vi "TR_Repair_TDMS_track.vi"(8 "error in (no error)":errorcluster, 10 "Parameters":T1, 11 "TDMS track":path) -> (0 "error out":errorcluster)   [LabVIEW 2018, in "Tracks Repair.lvlib"]
uses:
  Tracks Repair.lvlib
  SubVi's/Controls/CTL_Overlays_cluster.ctl
  SubVi's/Controls/CTL_Settings_cluster.ctl
  SubVi's/Controls/CTL_Histogram_parameters.ctl
  SubVi's/Controls/CTL_Filter_selector.ctl
  SubVi's/Controls/CTL_Acquisition_speed_selector.ctl
  SubVi's/Controls/CTL_Segmented_plot_parameters.ctl
  SubVi's/Controls/CTL_IO_params_cluster.ctl
  SubVi's/Controls/CTL_Conditions_Array.ctl
  SubVi's/Controls/CTL_Conditions_Cluster.ctl
  SubVi's/Controls/CTL_Condition_type.ctl
  SubVi's/Controls/CTL_Comparison_type.ctl
  SubVi's/Controls/CTL_Validity_check_criteria.ctl
  SubVi's/Controls/CTL_Response_info.ctl
  SubVi's/Controls/CTL_Condition_response_type.ctl
  SubVi's/Controls/CTL_Reponse_port_info.ctl
  SubVi's/Controls/CTL_Calibration_parameters.ctl
  SubVi's/Controls/CTL_Dispenser_calibration_info.ctl
  SubVi's/Controls/CTL_Post-processing_params.ctl
  SubVi's/Controls/CTL_Mouse_Draw_Params.ctl
  <vilib>/vision/Image Controls.llb/IMAQ Image.ctl
  SubVi's/Controls/CTL_Pixel_to_Zone_array.ctl
  SubVi's/Controls/CTL_Basic_cage_settings.ctl
  <userlib>/_OpenG.lib/md5/md5.llb/MD5 Message Digest (Hexadecimal String)__ogtk.vi
  <userlib>/_OpenG.lib/file/file.llb/Strip Path Extension - String__ogtk.vi
  Tracker.lvlib
panel:
  in  "Decimate?":bool
  out "Overlays cluster out":T2
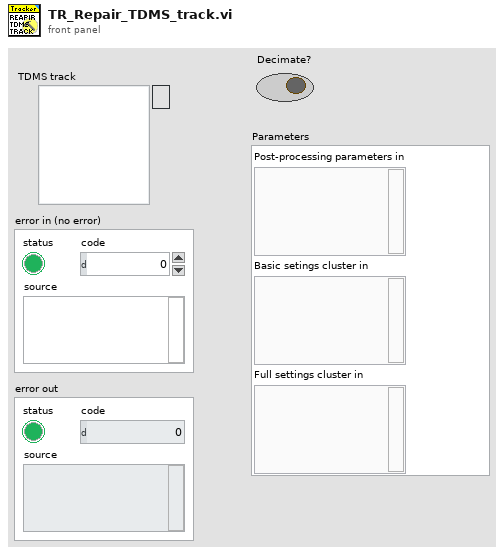
[diagram p1: front panel]
types:
  T1 = cluster{"Post-processing parameters in":variant, "Basic setings cluster in":variant, "Full settings cluster in":variant}
  T2 = typedef "Tracker.lvlib/CTL_Overlays_cluster.ctl" = cluster{"Time-coded track overlay (array)":u32[][], "Speed-coded track overlay (array)":u32[][], "Plain track overlay pixmap":u32[][], "Location density map image":u32[][], "Speed density map image":u32[][], "Location density map":dbl[][], "Speed density map":dbl[][]}
  T3 = enum16{"big-endian, network order", "native, host order", "little-endian"}
  T4 = enum16{"open", "open or create", "create or replace", "create", "open (read-only)"}
  T5 = typedef "Tracker.lvlib/CTL_Basic_cage_settings.ctl" = cluster{"Vert. offset":dbl, "Hor. offset":dbl, "Bridge swap":bool, "Twisted neck":bool, "Cage diam.":i32, "Magn.rot.":i32, "Acq. speed":dbl}
  T6 = typedef "Tracker.lvlib/CTL_Post-processing_params.ctl" = cluster{"Defragment TDMS? (F)":bool, "Start time (SW)":timestamp, "Start time (HW)":u32, "Data filtering":T7, "Mouse drawing parameters":T8, "Size of the image (480x480)":cluster{"X size":dbl, "Y size":dbl}, "Image ref. in":T9, "Calibration parameters":T10, "Pixel to zone":T12}
  T7 = typedef "Tracker.lvlib/CTL_Filter_selector.ctl" = cluster{"Filter type":enum16{"None", "Savitzky-Golay"}, "Length":i32, "Order":i32}
  T8 = typedef "Tracker.lvlib/CTL_Mouse_Draw_Params.ctl" = cluster{"Trace length, samples":u16, "Rainbow track":bool, "Rainbow track is speed":bool, "Bright mouse lineout":bool, "Colors array":u32[], "Pixels per mm":dbl}
  T9 = typedef "IMAQ Image.ctl" = refnum<image>
  T10 = typedef "Tracker.lvlib/CTL_Calibration_parameters.ctl" = cluster{"Timing calibration sw/hw":dbl, "True FPS":dbl, "True frame time, s":dbl, "Disp. calibration info":T11}
  T11 = typedef "Tracker.lvlib/CTL_Dispenser_calibration_info.ctl" = cluster{"Channel":u8, "Speed, µl per ms":dbl}[]
  T12 = typedef "Tracker.lvlib/CTL_Pixel_to_Zone_array.ctl" = i8[][]
  T13 = typedef "Tracker.lvlib/CTL_Settings_cluster.ctl" = cluster{"Defaults":cluster{"Default User":dbl, "VISA Resource Name ":string, "Histogram parameters":T14}, "Recording and saving":cluster{"Researcher name":string, "Name prefix":string, "Data post-processing":T7, "Stop at":dbl, "\"Stop at\" enabled":bool, "Default save folder path":path, "Acquisition FPS":T15}, "Geometry":T16, "IO parameters":T17, "Conditions presets array":T18, "Calibration parameters":T10, "Settings loaded OK":bool}
  T14 = typedef "Tracker.lvlib/CTL_Histogram_parameters.ctl" = cluster{"max":dbl, "min":dbl, "# bins":i32, "threshold":dbl, "thr. type":enum16{"higher accepted", "lower accepted"}}
  T15 = typedef "Tracker.lvlib/CTL_Acquisition_speed_selector.ctl" = enum16{"Max", "Optimal", "Eco"}
  T16 = typedef "Tracker.lvlib/CTL_Segmented_plot_parameters.ctl" = cluster{"Cage diameter, mm":u16, "Starting angle MIDFIELD":i16, "Starting angle BORDER":i16, "Radius, mm CENTER":u16, "Radius, mm MIDFIELD":u16, "N segments MIDFIELD":u8, "N segments BORDER":u8, "R-gap, mm":sgl, "Bridge swap":bool, "Bridge H. offset":sgl, "Bridge V. offset":sgl, "Twisted neck":bool, "Alt. magn. orientation":bool, "Sensor board size":enum16{"Small", "Large"}}
  T17 = typedef "Tracker.lvlib/CTL_IO_params_cluster.ctl" = cluster{"IO general config.":u16, "IO 1 configuration":u16, "IO 2 configuration":u16, "IO 3 configuration":u16, "IO 4 configuration":u16, "Activate ext. RS-232":u16, "IO inversion config.":u16, "Sync capability":u8}
  T18 = typedef "Tracker.lvlib/CTL_Conditions_Array.ctl" = T19[]
  T19 = typedef "Tracker.lvlib/CTL_Conditions_Cluster.ctl" = cluster{"Enabled":bool, "Name":string, "Specifier(s)":cluster{"Specifier enabled":bool, "Condition type":T20, "Comparison type":T21, "Value":dbl, "Validity criteria(s)":cluster{"V. check enabled":bool, "Criteria":T22, "Validity value":dbl}[]}[], "Response":T23, "Has been set":bool}
  T20 = typedef "Tracker.lvlib/CTL_Condition_type.ctl" = enum16{"Speed", "Zone", "Angle to wall"}
  T21 = typedef "Tracker.lvlib/CTL_Comparison_type.ctl" = enum16{"Less", "Less or Equal", "Equal", "Greater or Equal", "Greater", "Not Equal"}
  T22 = typedef "Tracker.lvlib/CTL_Validity_check_criteria.ctl" = enum16{"Running bout (seconds)", "Running bout (meters)"}
  T23 = typedef "Tracker.lvlib/CTL_Response_info.ctl" = cluster{"Response type":T24, "TTL port":T25, "TTL pulse length, ms":dbl}
  T24 = typedef "Tracker.lvlib/CTL_Condition_response_type.ctl" = enum16{"None", "Air puff", "Liquid reward"}
  T25 = typedef "Tracker.lvlib/CTL_Reponse_port_info.ctl" = enum16{"Port 1", "Port 2", "Port 3", "Port 4"}
  T26 = typedef "Tracker.lvlib/CTL_Cage_Coords_(arrays).ctl" = cluster{"R from center":dbl[], "sin(a)":dbl[], "Mouse Xc":dbl[], "Mouse Yc":dbl[], "X1-X2":dbl[], "Y1-Y2":dbl[], "Cage Xc":dbl[], "Cage Yc":dbl[], "Frame time, s":dbl}
  T27 = typedef "Tracker.lvlib/CTL_Animal_Coordinates_and_Speed_(arr).ctl" = cluster{"R from center":dbl[], "phi (mouse angular position in the cage)":dbl[], "alpha (mouse rot. angle)":dbl[], "X":dbl[], "Y":dbl[], "theta (from center towards mouse)":dbl[], "beta (cage rot. against mouse)":dbl[], "w (mouse angle to wall)":dbl[], "Speed (filtered)":dbl[], "Zone":i8[]}
  T28 = cluster{"Boolean Round":bool, "code":i32, "source":string}
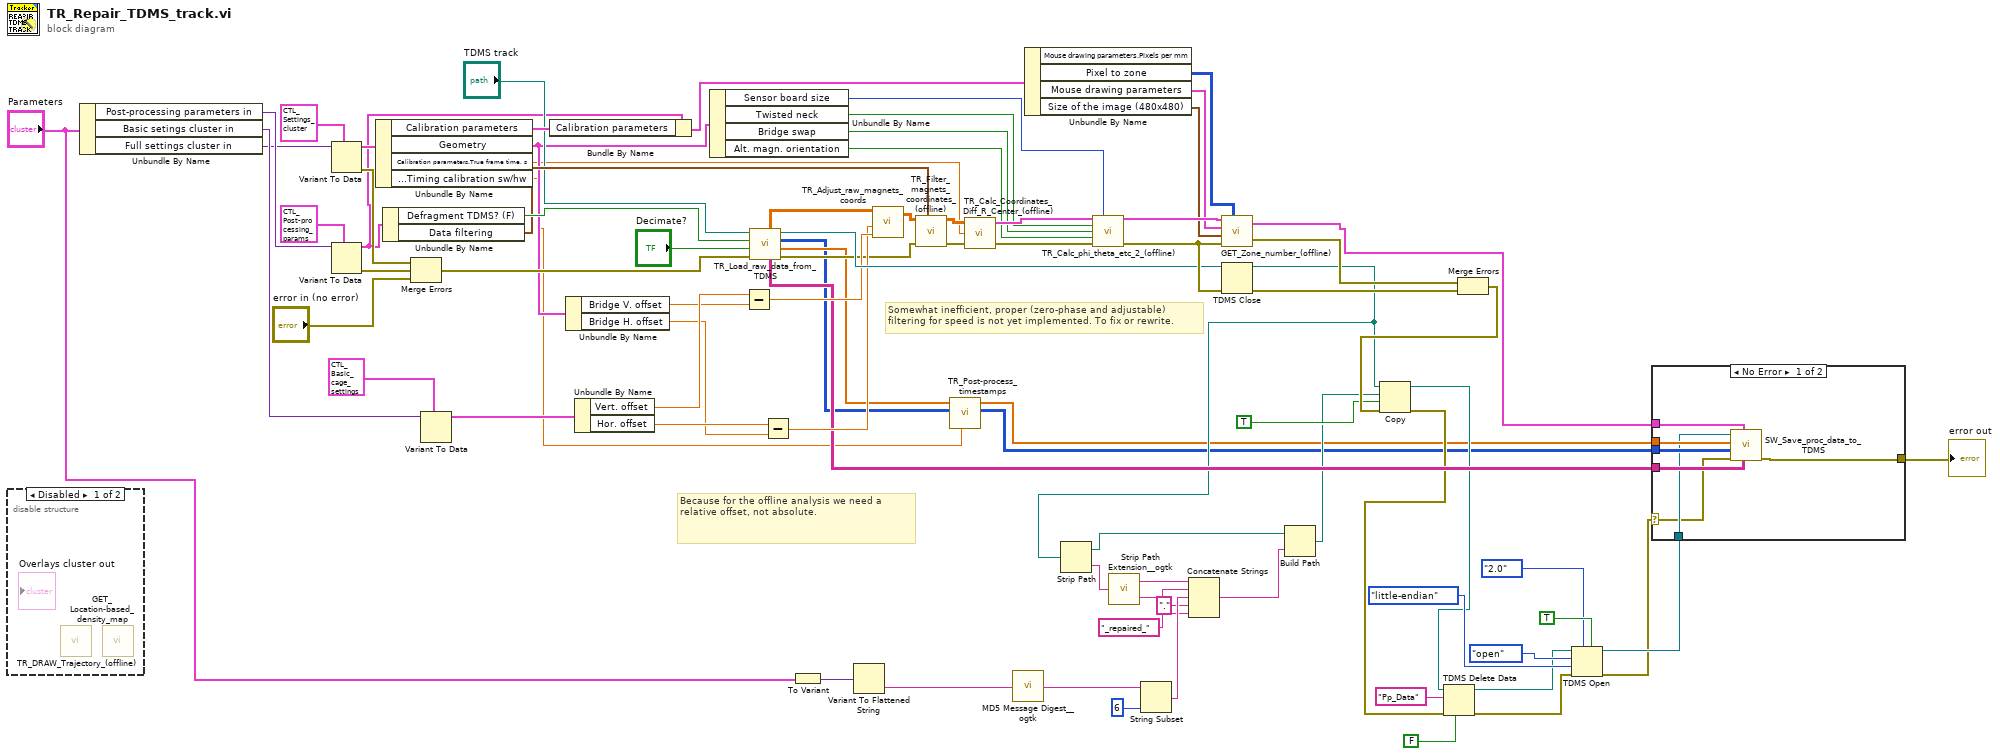
[diagram p0: block diagram]
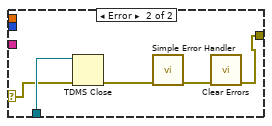
[diagram p2: hidden frame]
diagram:
  # "Because for the offline analysis we need a relative offset, not absolute."
  # "Somewhat inefficient, proper (zero-phase and adjustable) filtering for speed is not yet implemented. To fix or rewrite."
  n1 = disable-structure shown="Disabled" {
    frame Disabled {
      n2 = call "TR_DRAW_Trajectory_(offline).vi"() -> ()  [unwired: 13 in, 3 out]
      n3 = call "GET_Location-based_density_map.vi"() -> ()  [unwired: 13 in, 3 out]
    }
    frame Enabled {
    }
  }
  n4 = Unbundle By Name("Parameters") -> ("Post-processing parameters in"=w42:variant, "Basic setings cluster in"=w41:variant, "Full settings cluster in"=w40:variant)
  n5 = Variant To Data(type=T13 {"Defaults"={"Default User"=0.0, "VISA Resource Name "="", "Histogram parameters"={"max"=300.0, "min"=0.0, "# bins"=10, "threshold"=8.0, "thr. type"=enum."higher accepted"}}, "Recording and saving"={"Researcher name"="", "Name prefix"="", "Data post-processing"={"Filter type"=enum."None", "Length"=0, "Order"=0}, "Stop at"=0.0, "\"Stop at\" enabled"=FALSE, "Default save folder path"=path "", "Acquisition FPS"=enum."Max"}, "Geometry"={"Cage diameter, mm"=0, "Starting angle MIDFIELD"=0, "Starting angle BORDER"=0, "Radius, mm CENTER"=0, "Radius, mm MIDFIELD"=0, "N segments MIDFIELD"=0, "N segments BORDER"=0, "R-gap, mm"=0.0, "Bridge swap"=FALSE, "Bridge H. offset"=0.0, "Bridge V. offset"=0.0, "Twisted neck"=FALSE, "Alt. magn. orientation"=FALSE, "Sensor board size"=enum."Small"}, "IO parameters"={"IO general config."=0, "IO 1 configuration"=0, "IO 2 configuration"=0, "IO 3 configuration"=0, "IO 4 configuration"=0, "Activate ext. RS-232"=0, "IO inversion config."=0, "Sync capability"=0}, "Conditions presets array"=[], "Calibration parameters"={"Timing calibration sw/hw"=0.0, "True FPS"=0.0, "True frame time, s"=0.0, "Disp. calibration info"=[]}, "Settings loaded OK"=FALSE} ("Settings cluster"), Variant=w40) -> (data=w60:T13, error out=w58:errorcluster)  [unwired: 1 in]
  n6 = Variant To Data(type=T6 {"Defragment TDMS? (F)"=FALSE, "Start time (SW)"=timestamp(0 s since 1904-01-01), "Start time (HW)"=0, "Data filtering"={"Filter type"=enum."Savitzky-Golay", "Length"=41, "Order"=3}, "Mouse drawing parameters"={"Trace length, samples"=0, "Rainbow track"=FALSE, "Rainbow track is speed"=FALSE, "Bright mouse lineout"=FALSE, "Colors array"=[], "Pixels per mm"=0.0}, "Size of the image (480x480)"={"X size"=480.0, "Y size"=480.0}, "Image ref. in"=refnum, "Calibration parameters"={"Timing calibration sw/hw"=1.0, "True FPS"=80.0, "True frame time, s"=0.0125, "Disp. calibration info"=[]}, "Pixel to zone"=[]} ("Processing parameters"), Variant=w42) -> (data=w57:T6, error out=w56:errorcluster)  [unwired: 1 in]
  n7 = Unbundle By Name(w60) -> ("Calibration parameters"=w74:T10, "Geometry"=w49:T16, "Calibration parameters.True frame time, s"=w2:dbl, "Calibration parameters.Timing calibration sw/hw"=w1:dbl)
  n8 = Unbundle By Name(w57) -> ("Defragment TDMS? (F)"=w76:bool, "Data filtering"=w75:T7)
  n9 = Merge Errors(w58, w56, "error in (no error)") -> (w59:errorcluster)
  n10 = Variant To Data(type=T5 {"Vert. offset"=48.0, "Hor. offset"=0.0, "Bridge swap"=FALSE, "Twisted neck"=FALSE, "Cage diam."=325, "Magn.rot."=0, "Acq. speed"=100.01280589338842} ("Settings"), Variant=w41) -> (data=w50:T5)  [unwired: 1 in, 1 out]
  n11 = Bundle By Name(cluster=w57, "Calibration parameters"=w74) -> (w73:T6)
  n12 = Unbundle By Name(w49) -> ("Bridge V. offset"=w47:sgl, "Bridge H. offset"=w45:sgl)
  n13 = Unbundle By Name(w50) -> ("Vert. offset"=w48:dbl, "Hor. offset"=w46:dbl)
  n14 = Unbundle By Name(w49) -> ("Sensor board size"=w77:enum16{"Small", "Large"}, "Twisted neck"=w79:bool, "Bridge swap"=w78:bool, "Alt. magn. orientation"=w52:bool)
  n15 = Subtract(x=w48, y=w47) -> (x-y=w44:dbl)
  n16 = call "TR_Load_raw_data_from_TDMS.vi"("error in (no error)"=w59, "Decimate?"="Decimate?", "Defragment TDMS? (F)"=w76, "TDMS track ref. in"="TDMS track") -> ("error out"=w37:errorcluster, "SW timestamp"=w6:dbl[], "HW ts and Frame HW time"=w4:u32[][], "TDMS track ref. out"=w65:refnum<k34>, "TTL IO and Key"=w38:string[][], "Raw values"=w54:dbl[][])  [unwired: 2 in]
  n17 = Subtract(x=w46, y=w45) -> (x-y=w43:dbl)
  n18 = To Variant(anything="Parameters") -> (Variant=w26:variant)
  n19 = Variant To Flattened String(Variant=w26) -> (data string=w25:string)  [unwired: 1 out]
  n20 = call "TR_Adjust_raw_magnets_coords.vi"("Offset V."=w44, "Offset H."=w43, "Raw values in"=w54) -> ("Off-values out"=w53:dbl[][])  [unwired: 4 in]
  n21 = call "TR_Filter_magnets_coordinates_(offline).vi"("Data filtering"=w75, "error in (no error)"=w37, "Magnets raw coordinates in"=w53) -> ("error out"=w83:errorcluster, "Magnets filtered coordinates out"=w82:dbl[][])  [unwired: 7 in]
  n22 = call "TR_Post-process_timestamps.vi"("Timing calibration sw/hw"=w1, "HW timestamp and delta in"=w4, "SW timestamp in"=w6) -> ("HW timestamp and delta out"=w3:u32[][], "SW timestamp out"=w5:dbl[])  [unwired: 7 in]
  n23 = call "TR_Calc_Coordinates_Diff_R_Center_(offline).vi"("Error In"=w83, "Frame time, s"=w2, "Magnets coordinates in"=w82) -> ("Error Out"=w81:errorcluster, "Output cluster of data"=w80:T26)  [unwired: 1 in]
  n24 = call-poly <userlib>:"MD5 Message Digest__ogtk.vi"("Message"=w25) -> ("MD5 Message Digest"=w24:string)
  n25 = Unbundle By Name(w73) -> ("Pixel to zone"=w70:T12, "Mouse drawing parameters"=w71:T8, "Size of the image (480x480)"=w69:cluster{"X size":dbl, "Y size":dbl})  [unwired: 1 out]
  n26 = call "TR_Calc_phi_theta_etc_2_(offline).vi"("Input data cluster"=w80, "SB size"=w77, "Twisted neck"=w79, "Bridge swap"=w78, "Use alternative magnets orientation"=w52, "Error In"=w81) -> ("Animal coordinates cluster"=w72:T27, "Error out"=w66:errorcluster)  [unwired: 8 in]
  n27 = String Subset(string=w24, length (rest)=6 ("length (rest)")) -> (substring=w20:string)  [unwired: 1 in]
  n28 = call "GET_Zone_number_(offline).vi"("Animal coordinates cluster in"=w72, "Mouse drawing parameters"=w71, "Size of the image (480x480)"=w69, "error in (no error)"=w66, "Array of the pixel to zone correspondences"=w70) -> ("Animal coordinates cluster out"=w39:T27, "error out"=w62:T28)
  n29 = TDMS Close(8:w66, 11:w65) -> (0:w63:errorcluster, 3:w15:path)
  n30 = Strip Path(path=w15) -> (stripped path=w13:path, name=w28:string)
  n31 = call-poly <userlib>:"Strip Path Extension__ogtk.vi"("path"=w28) -> ("root"=w22:string, "extension"=w18:string)
  n32 = Concatenate Strings(w22, "_repaired_" ("string"), w20, "." ("string"), w18) -> (w16:string)
  n33 = Build Path(base path=w13, name or relative path=w16) -> (appended path=w14:path)
  n34 = Merge Errors(w62, w63) -> (w35:errorcluster)
  n35 = Copy(8:w35, 9:TRUE ("overwrite (F)"), 10:w14, 11:w15) -> (0:w12:errorcluster, 3:w10:path)  [unwired: 1 in, 1 out]
  n36 = TDMS Delete Data(6:FALSE ("keep empty group/channel? (T)"), 8:w12, 10:"Pp_Data" ("group name in"), 11:w10) -> (0:w11:errorcluster, 3:w9:path)  [unwired: 3 in]
  n37 = TDMS Open(5:TRUE ("create index file? (T)"), 7:enum16{"1.0", "2.0"}."2.0" ("file format version (2.0)"), 8:w11, 9:T3."little-endian" ("byte order (2:little-endian)"), 10:T4."open" ("operation (0:open)"), 11:w9) -> (0:w19:errorcluster, 3:w29:refnum<k34>)  [unwired: 1 in]
  n38 = case shown="No Error" w19 {
    selector: w19 -> [w84 w94]
    tunnel: w39 -> [w90 _]
    tunnel: w38 -> [w89 _]
    tunnel: w3 -> [w88 _]
    tunnel: w5 -> [w87 _]
    tunnel: [w86 w91] -> w36
    tunnel: w29 -> [w85 w95]
    frame No Error {
      n39 = call "SW_Save_proc_data_to_TDMS.vi"("TTL IO and Key in"=w89, "Processed animal coordinates and speed"=w90, "error in (no error)"=w84, "HW timestamp and delta in"=w88, "SW timestamp in"=w87, "TDMS file ref. in"=w85) -> ("error out"=w86:errorcluster)  [unwired: 5 in]
    }
    frame Error {
      n40 = TDMS Close(8:w94, 11:w95) -> (0:w93:errorcluster)  [unwired: 1 out]
      n41 = call <vilib>:"Simple Error Handler.vi"("error in (no error)"=w93) -> ("error out"=w92:errorcluster)  [unwired: 4 in, 4 out]
      n42 = call <vilib>:"Clear Errors.vi"("error in (no error)"=w92) -> ("error out"=w91:errorcluster)  [unwired: 5 in, 1 out]
    }
  }
  "error out" <- w36
